vi "Rearrange 2D Data.vi"(8 "error in (no error)":errorcluster, 10 "All Headers Order":string[](array[string]), 11 "2D Data with Headers In":string[][](array[string])) -> (0 "error out":errorcluster, 3 "2D Data Out without Headers[]":string[][](array[string]))   [LabVIEW 2014, in "SLL Spreadsheet.lvlib" / "SLL CSV Logger.lvclass"]
uses:
  SLL CSV Logger.lvclass
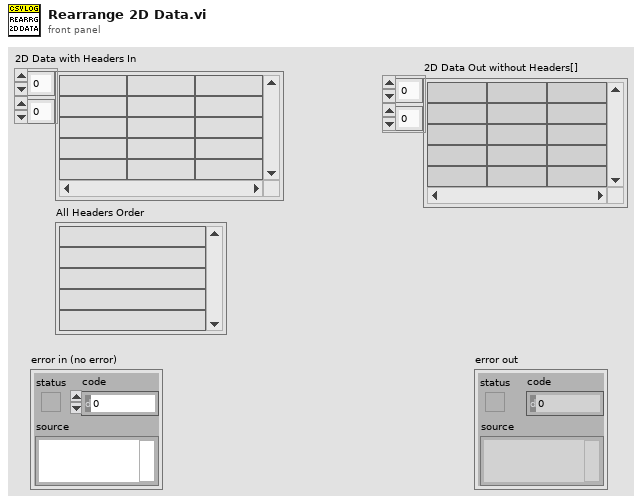
[diagram p1: front panel]
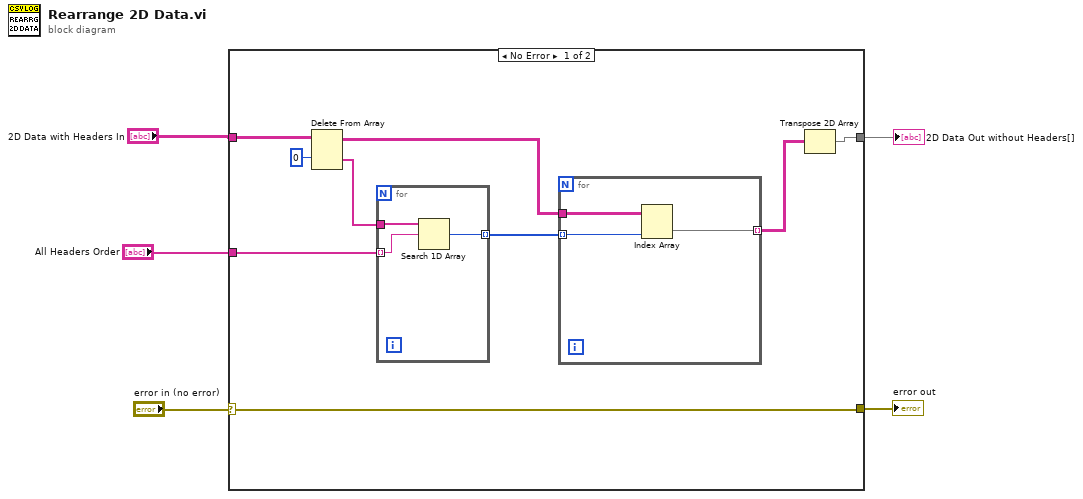
[diagram p0: block diagram]
diagram:
  n1 = case shown="No Error" "error in (no error)" {
    selector: "error in (no error)" -> [w14 w22]
    tunnel: [w14 w22] -> w4
    tunnel: "2D Data with Headers In" -> [w9 w21]
    tunnel: [w7 w21] -> w2
    tunnel: "All Headers Order" -> [w12 _]
    frame No Error {
      n2 = Delete From Array(array=w9, index (row)=0) -> (deleted portion=w11:string[], array with subset deleted=w6:string[][])  [unwired: 2 in]
      n3 = for {
        tunnel: w12 -> [w19] mode=indexing
        tunnel: w11 -> [w20]
        tunnel: [w18] -> w10 mode=indexing
        n4 = Search 1D Array(1D array=w20, element=w19) -> (index of element=w18:i32)  [unwired: 1 in]
      }
      n5 = for {
        tunnel: w10 -> [w16] mode=indexing
        tunnel: w6 -> [w17]
        tunnel: [w15] -> w8 mode=indexing
        n6 = Index Array(array=w17, index (col)=w16) -> (element=w15:string[])  [unwired: 1 in]
      }
      n7 = Transpose 2D Array(2D array=w8) -> (transposed array=w7:string[][])
    }
    frame Error {
    }
  }
  "error out" <- w4
  "2D Data Out without Headers[]" <- w2
